vi "Test ALl BG.vi"() -> ()   [LabVIEW 2020]
panel:
  in  "Range":cluster{"Numeric":dbl, "Numeric":dbl}(slide)={"Numeric"=0.0, "Numeric"=1.2307692307692308} scale=0.0..100.0 scale format="%#_2f"
  in  "String":string
  out "XY Graph":cluster{"X":dbl, "Y":dbl}[](graph)
  in  "Tree":string(tree)
  in  "Multicolumn Listbox":i32(listbox)
  in  "Boolean":bool
  out "Array":string[](array[string])
  out "Control Value:Get All":cluster{"Name":string, "Variant Data":variant}[](array[cluster])
  out "Waveform Chart 2":dbl(graph)
  out "Waveform Chart":dbl(graph)
  in  "Stop":bool
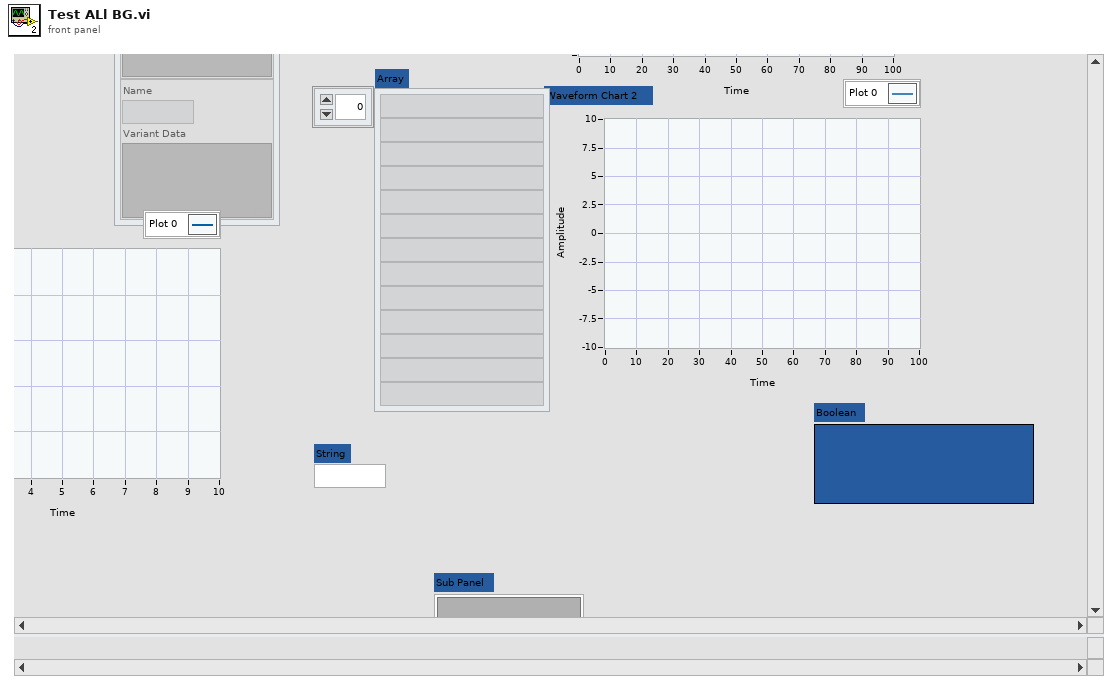
[diagram p1: front panel]
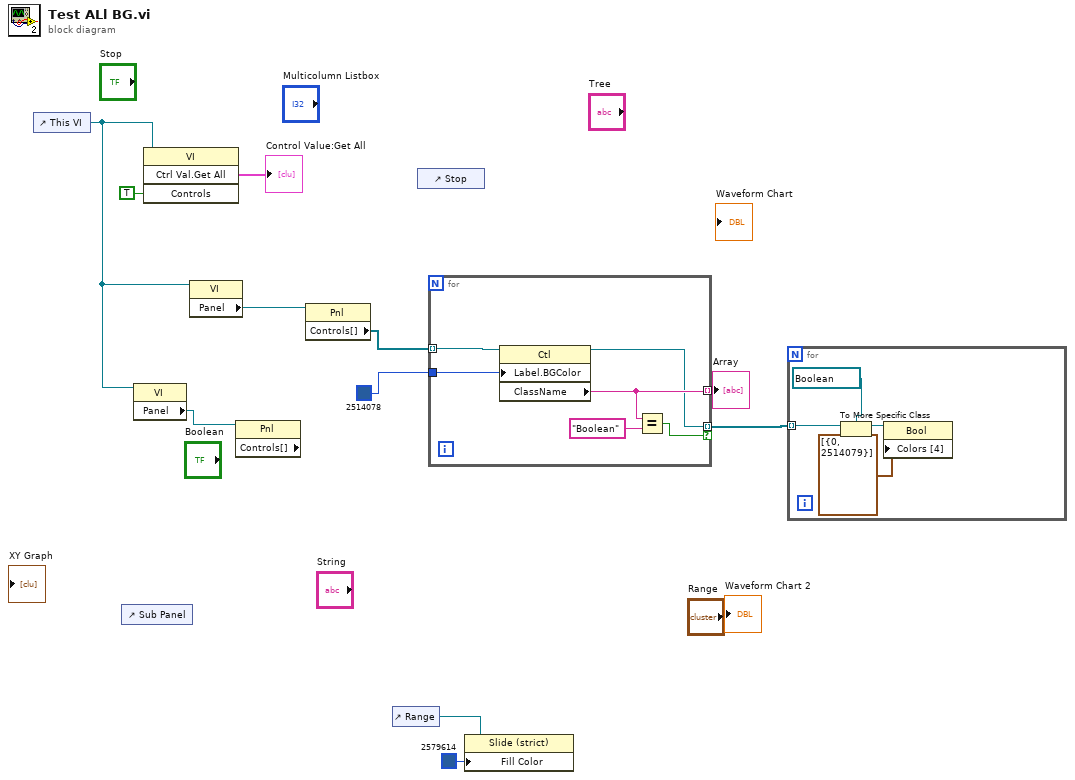
[diagram p0: block diagram]
diagram:
  n1 = control-ref of="This VI"() -> (w7:refnum<vi>)
  n2 = control-ref of="Sub Panel"() -> ()  [unwired: 1 out]
  n3 = property class="VI"(reference=w7) -> ("Panel"=w5:refnum<vi>)  [unwired: 1 in, 2 out]
  n4 = invoke class="VI" method="Ctrl Val.Get All"(reference=w7, "Controls"=TRUE) -> ("Get All Control Values Variant"=→"Control Value:Get All":cluster{"Name":string, "Variant Data":variant}[])  [unwired: 2 in, 3 out]
  n5 = property class="VI"(reference=w7) -> ("Panel"=w6:refnum<vi>)  [unwired: 1 in, 2 out]
  n6 = property class="Pnl" props=["Controls[]"](reference=w5) -> ()  [unwired: 1 in, 3 out]
  n7 = property class="Pnl"(reference=w6) -> ("Controls[]"=w9:refnum<vi>[])  [unwired: 1 in, 2 out]
  n8 = control-ref of="Range"() -> (w2:refnum<vi>)
  n9 = control-ref of="Stop"() -> ()  [unwired: 1 out]
  n10 = for {
    tunnel: w9 -> [w17] mode=indexing
    tunnel: u32 2514078 -> [w16]
    tunnel: [w15] -> w4 mode=indexing
    tunnel: [w13] -> w3 mode=indexing if=w12
    n11 = property class="Ctl"(reference=w17, "Label.BGColor"=w16) -> (reference out=w13:refnum<vi>, "ClassName"=w15:string)  [unwired: 1 in, 1 out]
    n12 = Equal?(x=w15, y="Boolean") -> (x = y?=w12:bool)
  }
  "Array" <- w4
  n13 = property class="Slide (strict)"(reference=w2, "Fill Color"=u32 2579614 ("Slider Colors:BG Color")) -> ()  [unwired: 1 in, 2 out]
  n14 = for {
    tunnel: w3 -> [w21] mode=indexing
    n15 = To More Specific Class(target class=refnum<vi> refnum ("Stop"), reference=w21) -> (specific class reference=w19:refnum<vi>)  [unwired: 1 in, 1 out]
    n16 = property class="Bool"(reference=w19, "Colors [4]"=cluster{u32, u32}[] [{0, 2514079}]) -> ()  [unwired: 1 in, 2 out]
  }
